vi "ma_SML OBW.vi"(8 "error in (no error)":errorcluster, 9 "% occupied BW":dbl=99.0 format="%.2f", 10 "spectral info":T1 {"window" items=["Rectangle"=0, "Hanning"=1, "Hamming"=2, "Blackman-Harris"=3, "Exact Blackman"=4, "Blackman"=5, "Flat Top"=6, "4 Term B-Harris "=7, "7 Term B-Harris"=8, "Low Sidelobe"=9, "Blackman Nuttall"=11, "Triangle"=30, "Bartlett-Hanning"=31, "Bohman"=32, "Parzen"=33, "Welch"=34, "Kaiser"=60, "Dolph-Chebyshev"=61, "Gaussian"=62]}, 11 "power spectrum":T2={"f0"=0.0, "df"=1.0, "spectrum"=[]} {"spectrum" format="%.2f"; "df" format="%.2f"; "f0" format="%.2f"}) -> (0 "error out":errorcluster, 1 "fh [Hz]":dbl format="%.2f", 2 "fl [Hz]":dbl format="%.2f", 3 "occupied BW [Hz]":dbl format="%.2f")   [LabVIEW 2020, in "NI_MAPro.lvlib"]
uses:
  NI_MAPro.lvlib
  ma_sml_Spectrum Cluster (real).ctl
  ma_sml_Spectral Info.ctl
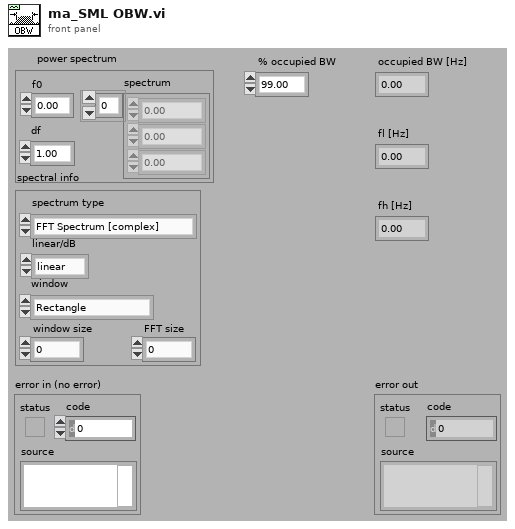
[diagram p1: front panel]
types:
  T1 = typedef "NI_MAPro.lvlib/ma_sml_Spectral Info.ctl" = cluster{"spectrum type":enum16{"FFT Spectrum [complex]", "Amplitude [Magnitude]", "Power [Magnitude^2]", "Cross Spectrum [complex]", "Frequency Response [Complex]"}, "linear/dB":enum16{"linear", "dB"}, "window":u16, "window size":i32, "FFT size":i32}
  T2 = typedef "NI_MAPro.lvlib/ma_sml_Spectrum Cluster (real).ctl" = cluster{"f0":dbl, "df":dbl, "spectrum":dbl[]}
  T3 = enum16{"FFT Spectrum [complex]", "Amplitude [Magnitude]", "Power [Magnitude^2]", "Cross Spectrum [complex]", "Frequency Response [Complex]"}
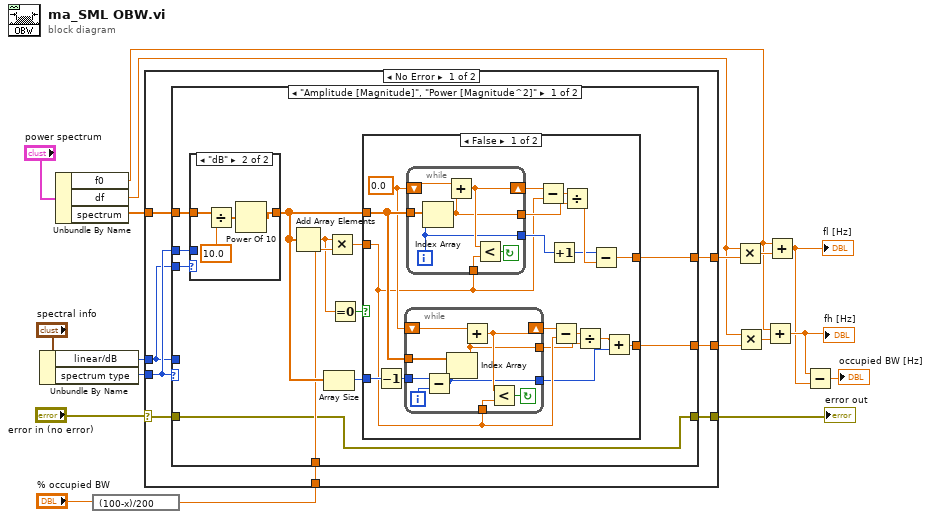
[diagram p0: block diagram]
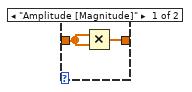
[diagram p3: hidden frame]
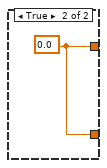
[diagram p4: hidden frame]
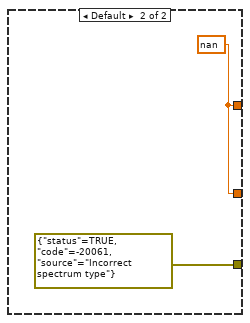
[diagram p5: hidden frame]
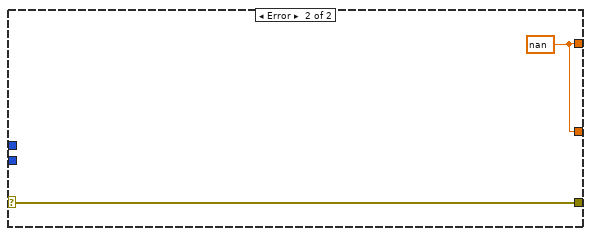
[diagram p6: hidden frame]
diagram:
  n1 = Unbundle By Name("spectral info") -> ("linear/dB"=w14:enum16{"linear", "dB"}, "spectrum type"=w15:T3)
  n2 = Unbundle By Name("power spectrum") -> ("f0"=w4:dbl, "df"=w5:dbl, "spectrum"=w12:dbl[])
  n3 = expression code="(100-x)/200"("% occupied BW") -> (w10:dbl)
  n4 = case shown="No Error" "error in (no error)" {
    selector: "error in (no error)" -> [w19 w87]
    tunnel: [w26 w87] -> w17
    tunnel: w15 -> [w25 _]
    tunnel: w14 -> [w20 _]
    tunnel: w12 -> [w24 _]
    tunnel: w10 -> [w23 _]
    tunnel: [w22 w86] -> w6
    tunnel: [w21 w86] -> w7
    frame No Error {
      n5 = case shown="\"Amplitude [Magnitude]\", \"Power [Magnitude^2]\"" w25 {
        tunnel: w20 -> [_ _]
        tunnel: [w27 errorcluster {"status"=TRUE, "code"=-20061, "source"="Incorrect spectrum type"} ("error IO")] -> w26
        tunnel: w25 -> [w38 _]
        tunnel: w24 -> [w37 _]
        tunnel: w23 -> [w35 _]
        tunnel: [w34 w84] -> w22
        tunnel: [w33 w84] -> w21
        tunnel: w20 -> [w28 _]
        tunnel: w19 -> [w27 _]
        frame "Amplitude [Magnitude]", "Power [Magnitude^2]" {
          n6 = case shown="\"dB\"" w28 {
            tunnel: w38 -> [w41 _]
            tunnel: w37 -> [w40 w46]
            tunnel: [w39 w48] -> w36
            frame "linear", Default {
              n7 = case shown="\"Power [Magnitude^2]\", Default" w41 {
                tunnel: w40 -> [w43 w44]
                tunnel: [w42 w44] -> w39
                frame "Amplitude [Magnitude]" {
                  n8 = Multiply(x=w43, y=w43) -> (x*y=w42:dbl[])
                }
                frame "Power [Magnitude^2]", Default {
                }
              }
            }
            frame "dB" {
              n9 = Divide(x=w46, y=10.0 ("Occupied BW [Hz]")) -> (x/y=w47:dbl[])
              n10 = Power Of 10(x=w47) -> (10^x=w48:dbl[])
            }
          }
          n11 = Add Array Elements(numeric array=w36) -> (sum=w32:dbl)
          n12 = Array Size(array=w36) -> (size(s)=w29:i32)
          n13 = Multiply(x=w32, y=w35) -> (x*y=w30:dbl)
          n14 = Equal To 0?(x=w32) -> (x = 0?=w31:bool)
          n15 = case shown="False" w31 {
            tunnel: [w60 w83] -> w34
            tunnel: [w50 w83] -> w33
            tunnel: w36 -> [w66 _]
            tunnel: w30 -> [w54 _]
            tunnel: w29 -> [w64 _]
            frame False {
              w65 = 0.0 ("Occupied BW [Hz]")
              n16 = Decrement(x=w64) -> (x-1=w55:i32)
              n17 = while {
                tunnel: [w74] -> w49
                tunnel: [w75] -> w52
                tunnel: w54 -> [w76]
                tunnel: w55 -> [w80]
                shift-left: w65 -> [w79]
                shift-right: [w78] -> w56
                tunnel: w66 -> [w81]
                i -> [w82]
                stop <- w77 continue-if-true
                n18 = Subtract(x=w80, y=w82) -> (x-y=w74:i32)
                n19 = Index Array(array=w81, index=w74) -> (element=w75:dbl)
                n20 = Add(x=w79, y=w75) -> (x+y=w78:dbl)
                n21 = Less?(x=w78, y=w76) -> (x < y?=w77:bool)
              }
              n22 = while {
                tunnel: w54 -> [w67]
                tunnel: [w68] -> w58
                tunnel: [w69] -> w61
                shift-left: w65 -> [w73]
                shift-right: [w70] -> w63
                tunnel: w66 -> [w72]
                i -> [w68]
                stop <- w71 continue-if-true
                n23 = Index Array(array=w72, index=w68) -> (element=w69:dbl)
                n24 = Add(x=w73, y=w69) -> (x+y=w70:dbl)
                n25 = Less?(x=w70, y=w67) -> (x < y?=w71:bool)
              }
              n26 = Subtract(x=w63, y=w54) -> (x-y=w62:dbl)
              n27 = Increment(x=w58) -> (x+1=w57:i32)
              n28 = Subtract(x=w56, y=w54) -> (x-y=w53:dbl)
              n29 = Divide(x=w62, y=w61) -> (x/y=w59:dbl)
              n30 = Divide(x=w53, y=w52) -> (x/y=w51:dbl)
              n31 = Subtract(x=w57, y=w59) -> (x-y=w60:dbl)
              n32 = Add(x=w51, y=w49) -> (x+y=w50:dbl)
            }
            frame True {
              w83 = 0.0 ("Occupied BW [Hz]")
            }
          }
        }
        frame Default {
          w84 = nan ("Occupied BW [Hz]")
        }
      }
    }
    frame Error {
      w86 = nan ("Occupied BW [Hz]")
    }
  }
  "error out" <- w17
  n33 = Multiply(x=w5, y=w6) -> (x*y=w9:dbl)
  n34 = Multiply(x=w5, y=w7) -> (x*y=w8:dbl)
  n35 = Add(x=w4, y=w8) -> (x+y=w2:dbl)
  "fh [Hz]" <- w2
  n36 = Add(x=w4, y=w9) -> (x+y=w1:dbl)
  "fl [Hz]" <- w1
  n37 = Subtract(x=w2, y=w1) -> (x-y=→"occupied BW [Hz]":dbl)
